vi "primero.vi"(2 "a":dbl, 3 "b":dbl, 4 "c":dbl) -> (0 "x":dbl, 1 "y":dbl)   [LabVIEW 2012]
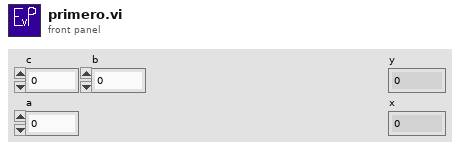
[diagram p1: front panel]
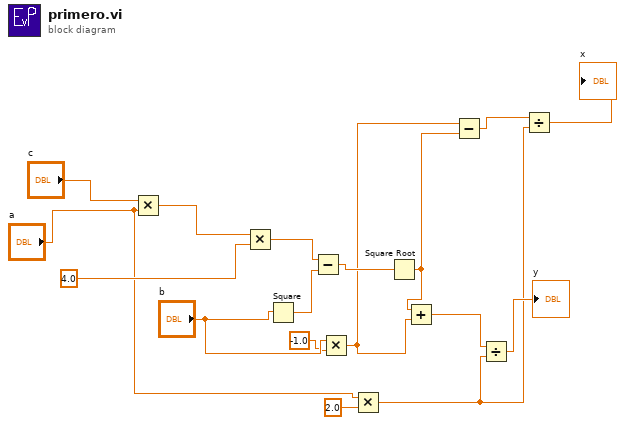
[diagram p0: block diagram]
diagram:
  n1 = Multiply(x="c", y="a") -> (x*y=w15:dbl)
  n2 = Multiply(x=w15, y=4.0) -> (x*y=w14:dbl)
  n3 = Square(x="b") -> (x^2=w13:dbl)
  n4 = Subtract(x=w14, y=w13) -> (x-y=w12:dbl)
  n5 = Multiply(x="b", y=-1.0 ("x")) -> (x*y=w3:dbl)
  n6 = Multiply(x="a", y=2.0) -> (x*y=w7:dbl)
  n7 = Square Root(x=w12) -> (sqrt(x)=w2:dbl)
  n8 = Add(x=w2, y=w3) -> (x+y=w11:dbl)
  n9 = Subtract(x=w3, y=w2) -> (x-y=w1:dbl)
  n10 = Divide(x=w11, y=w7) -> (x/y=→"y":dbl)
  n11 = Divide(x=w1, y=w7) -> (x/y=→"x":dbl)
